vi "NOVO Intezitet Senzora.vi"() -> ()   [LabVIEW 2017]
uses:
  <vilib>/Waveform/WDTOps.llb/WDT Index Channel DBL.vi
panel:
  in  "Tab Control":enum32{"LIVE DATA", "Podesavanja"}(tab)
  out "Inteziteti ACC 1":waveform(dbl)(graph)
  out "Inteziteti ACC 2":waveform(dbl)(graph)
  out "Inteziteti ACC 3":waveform(dbl)(graph)
  out "TRENUTNI SIGNALI":dynamicdata(graph) caption="TRENUTNI SIGNALI !!!!"
  out "Iter":i32
  in  "File Name":string="LIVE_DATA"
  in  "Ponavljanja":i32=20
  out "Maximum":dbl
  out "Intezitet":dbl[](array[numeric])
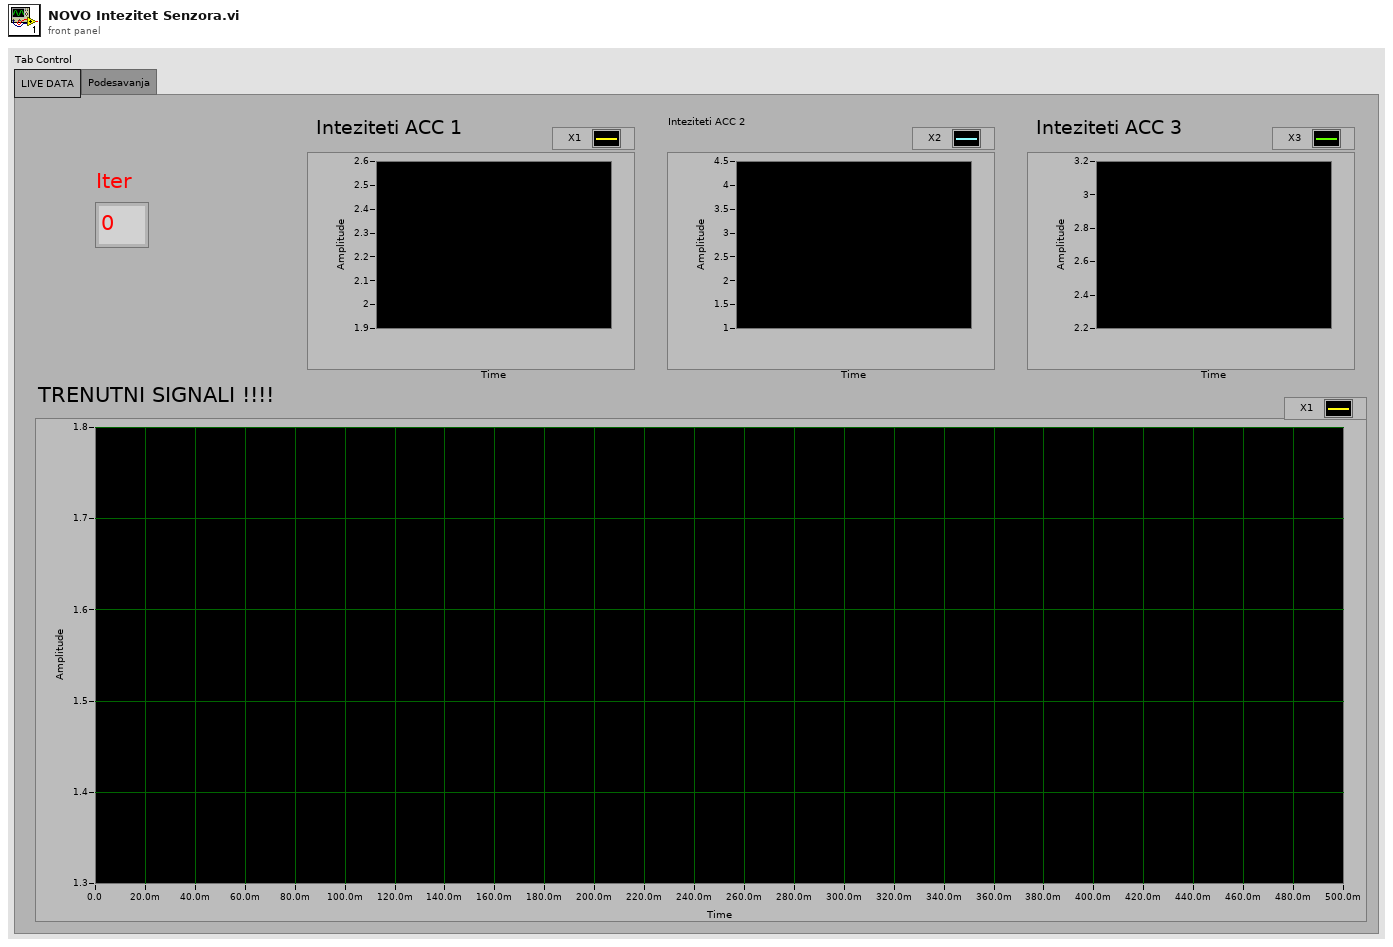
[diagram p1: front panel]
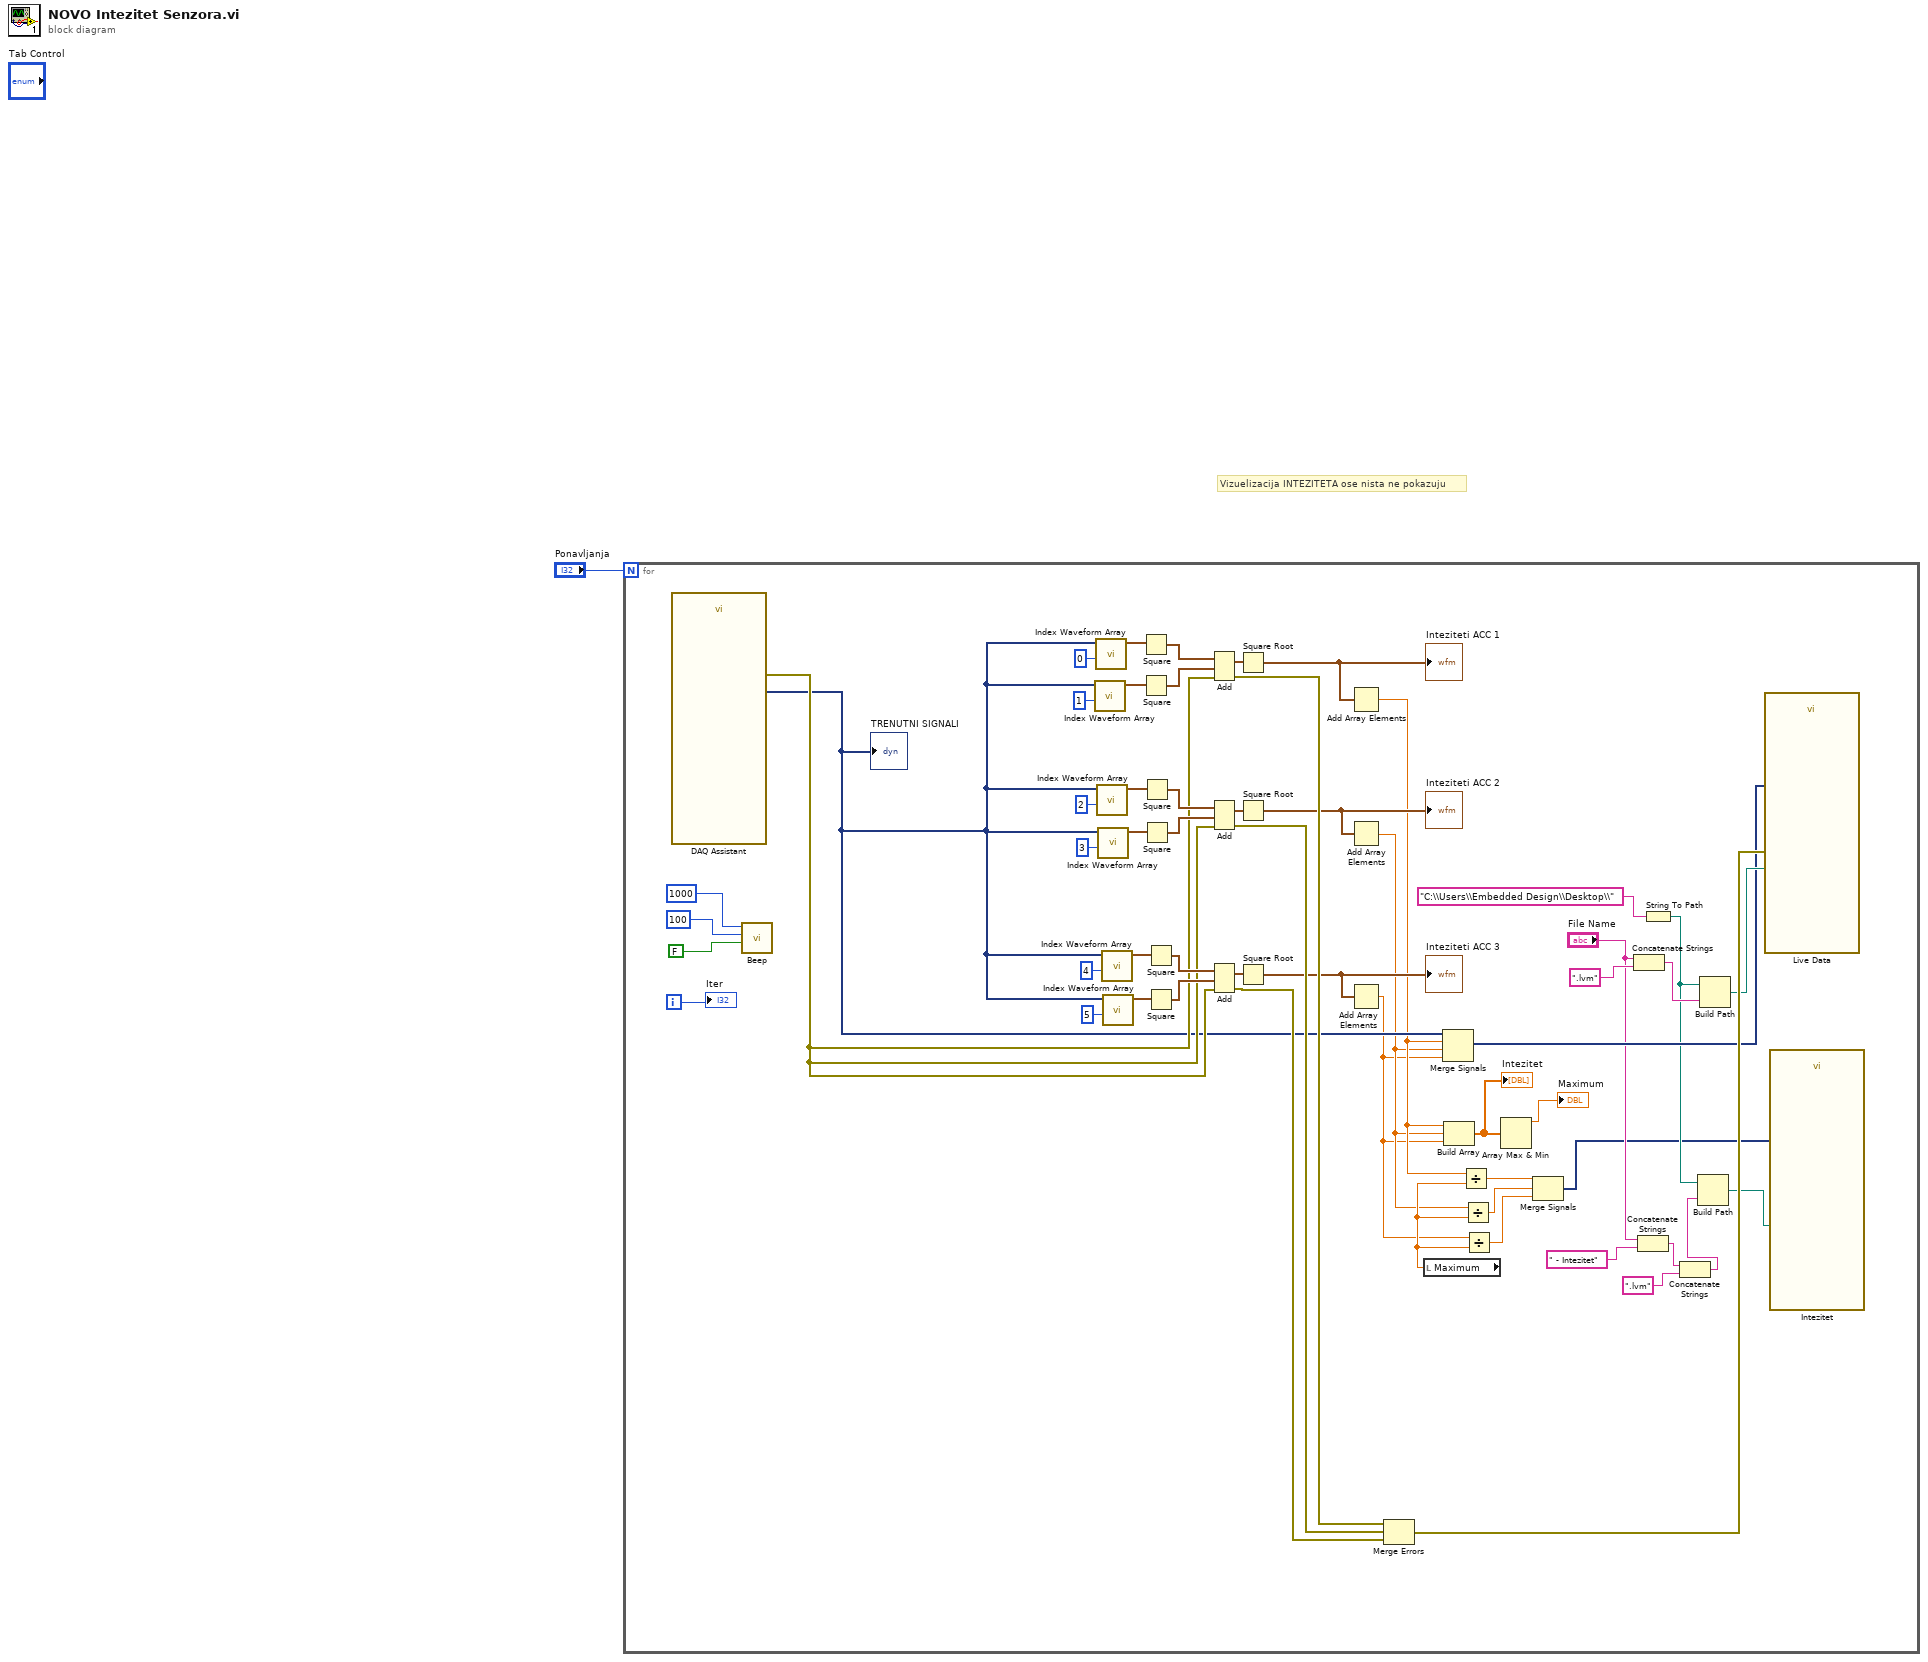
[diagram p0: block diagram]
diagram:
  # "Vizuelizacija INTEZITETA ose nista ne pokazuju"
  n1 = for {
    N: "Ponavljanja" -> [_]
    i -> [w21]
    n2 = call "DAQ Assistant"() -> ("data"=w6:dynamicdata, "error out"=w28:errorcluster)  [unwired: 16 in, 2 out]
    "TRENUTNI SIGNALI" <- w6
    n3 = call <vilib>:"Beep.vi"("use system alert? (T)"=FALSE, "duration (msec)"=u32 100, "frequency (Hz)"=u32 1000) -> ()  [unwired: 9 in]
    n4 = call-poly <vilib>:"Index Waveform Array.vi"("index"=1, "waveform array"=w6) -> ("waveform"=w42:waveform(dbl))  [unwired: 8 in, 1 out]
    n5 = call-poly <vilib>:"Index Waveform Array.vi"("index"=0, "waveform array"=w6) -> ("waveform"=w43:waveform(dbl))  [unwired: 8 in, 1 out]
    n6 = call-poly <vilib>:"Index Waveform Array.vi"("index"=2, "waveform array"=w6) -> ("waveform"=w41:waveform(dbl))  [unwired: 8 in, 1 out]
    n7 = call-poly <vilib>:"Index Waveform Array.vi"("index"=3, "waveform array"=w6) -> ("waveform"=w40:waveform(dbl))  [unwired: 8 in, 1 out]
    n8 = call-poly <vilib>:"Index Waveform Array.vi"("index"=4, "waveform array"=w6) -> ("waveform"=w39:waveform(dbl))  [unwired: 8 in, 1 out]
    n9 = call-poly <vilib>:"Index Waveform Array.vi"("index"=5, "waveform array"=w6) -> ("waveform"=w38:waveform(dbl))  [unwired: 8 in, 1 out]
    n10 = Square(x=w43) -> (x^2=w37:waveform(dbl))
    n11 = Square(x=w42) -> (x^2=w36:waveform(dbl))
    n12 = Square(x=w41) -> (x^2=w35:waveform(dbl))
    n13 = Square(x=w40) -> (x^2=w34:waveform(dbl))
    n14 = Square(x=w39) -> (x^2=w33:waveform(dbl))
    n15 = Square(x=w38) -> (x^2=w32:waveform(dbl))
    n16 = Add(1:w36, 2:w37, 4:w28) -> (0:w31:waveform(dbl), 3:w27:errorcluster)
    n17 = Add(1:w34, 2:w35, 4:w28) -> (0:w30:waveform(dbl), 3:w26:errorcluster)
    n18 = Add(1:w32, 2:w33, 4:w28) -> (0:w29:waveform(dbl), 3:w25:errorcluster)
    n19 = Square Root(x=w31) -> (sqrt(x)=w5:waveform(dbl))
    "Inteziteti ACC 1" <- w5
    n20 = Square Root(x=w30) -> (sqrt(x)=w24:waveform(dbl))
    "Inteziteti ACC 2" <- w24
    n21 = Square Root(x=w29) -> (sqrt(x)=w23:waveform(dbl))
    "Inteziteti ACC 3" <- w23
    n22 = Add Array Elements(numeric array=w5) -> (sum=w4:dbl)
    n23 = Add Array Elements(numeric array=w24) -> (sum=w3:dbl)
    n24 = Add Array Elements(numeric array=w23) -> (sum=w2:dbl)
    n25 = Merge Errors(w27, w26, w25) -> (w54:errorcluster)
    n26 = local read "Maximum"() -> (w9:dbl)
    n27 = Merge Signals(w6, w4, w3, w2) -> (w22:dynamicdata)
    n28 = Build Array(w4, w3, w2) -> (w8:dbl[])
    "Intezitet" <- w8
    n29 = Divide(x=w4, y=w9) -> (x/y=w12:dbl)
    n30 = Divide(x=w3, y=w9) -> (x/y=w13:dbl)
    n31 = Divide(x=w2, y=w9) -> (x/y=w11:dbl)
    n32 = Array Max & Min(array=w8) -> (max value=→"Maximum":dbl)  [unwired: 3 out]
    n33 = Merge Signals(w12, w13, w11) -> (w10:dynamicdata)
    n34 = Concatenate Strings("File Name", ".lvm" ("name or relative path")) -> (w50:string)
    n35 = Concatenate Strings("File Name", " - Intezitet" ("name or relative path")) -> (w18:string)
    n36 = String To Path(string="C:\\Users\\Embedded Design\\Desktop\\") -> (path=w16:path)
    n37 = Concatenate Strings(w18, ".lvm" ("name or relative path")) -> (w15:string)
    n38 = Build Path(base path=w16, name or relative path=w15) -> (appended path=w14:path)
    n39 = Build Path(base path=w16, name or relative path=w50) -> (appended path=w53:path)
    n40 = call "Live Data"("Signals"=w22, "error in (no error)"=w54, "Filename"=w53) -> ()  [unwired: 14 in, 3 out]
    n41 = call "Intezitet"("Signals"=w10, "Filename"=w14) -> ()  [unwired: 15 in, 3 out]
    "Iter" <- w21
  }
